vi "Remove Tag from TagsArray by ID.vi"(9 "Input TagsArray":refnum<class "Tag.lvclass">[](array[class]), 10 "Tag.lvclass":refnum<class "Tag.lvclass">) -> (1 "Output TagsArray":refnum<class "Tag.lvclass">[](array[class]))   [LabVIEW 2014]
doc: "Purpose of this VI is to remove an individual Tag object from an array of Tag objects whose ID equals input Tag object"
uses:
  Tag.lvclass
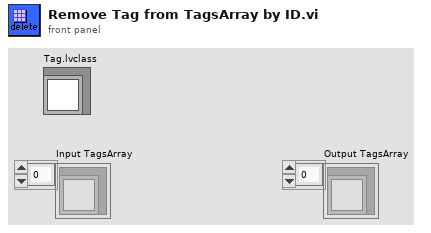
[diagram p1: front panel]
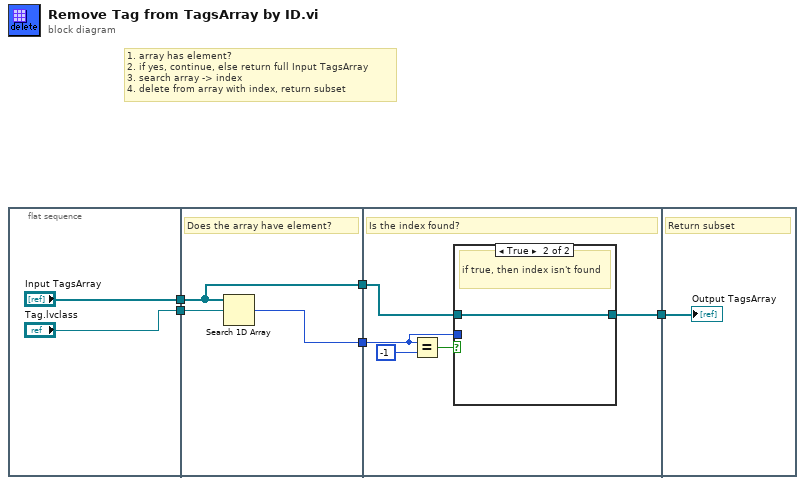
[diagram p0: block diagram]
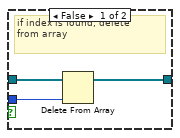
[diagram p2: hidden frame]
diagram:
  # "1. array has element?\n2. if yes, continue, else return full Input TagsArray\n3. search array -> index\n4. delete from array with index, return subset"
  n1 = flat-sequence {
    tunnel: ["Input TagsArray"] -> w5
    tunnel: ["Tag.lvclass"] -> w4
    tunnel: w5 -> [w8]
    tunnel: w4 -> [w10]
    tunnel: [w9] -> w3
    tunnel: [w8] -> w2
    tunnel: w3 -> [w11]
    tunnel: w2 -> [w13]
    tunnel: [w12] -> w1
    tunnel: w1 -> [w20]
    frame #0 {
    }
    frame #1 {
      # "Does the array have element?"
      n2 = Search 1D Array(1D array=w8, element=w10) -> (index of element=w9:i32)  [unwired: 1 in]
    }
    frame #2 {
      # "Is the index found?"
      n3 = Equal?(x=w11, y=-1) -> (x = y?=w14:bool)
      n4 = case shown="True" w14 {
        tunnel: w13 -> [w18 w19]
        tunnel: [w16 w19] -> w12
        tunnel: w11 -> [w17 _]
        frame False {
          # "if index is found, delete \nfrom array"
          n5 = Delete From Array(array=w18, index=w17) -> (array with subset deleted=w16:refnum<class "Tag.lvclass">[])  [unwired: 1 in, 1 out]
        }
        frame True {
          # "if true, then index isn't found"
        }
      }
    }
    frame #3 {
      # "Return subset"
      "Output TagsArray" <- w20
    }
  }
